vi "Turn Off all Chan.vi"(8 "error in (no error)":errorcluster, 11 "3300 in":refnum<class "3300.lvclass">) -> (0 "error out":errorcluster, 3 "3300 out":refnum<class "3300.lvclass">)   [LabVIEW 2019, in "3300.lvlib" / "3300.lvclass"]
uses:
  Library/3300.lvclass
  C:/Users/Public/Documents/Development/builds/Instruments/Electronic Load.lvlibp/Library/Electronic Load.lvclass
  builds/Instruments/Electronic Load.lvlibp/Custom Controls/E-Load Mode.ctl
  builds/Instruments/Electronic Load.lvlibp/Accessors/Trigger/Read Pulse Enable.vi
  builds/Instruments/Electronic Load.lvlibp/Accessors/Trigger/Read All Pulse.vi
  builds/Instruments/Electronic Load.lvlibp/Library/Electronic Load.lvclass
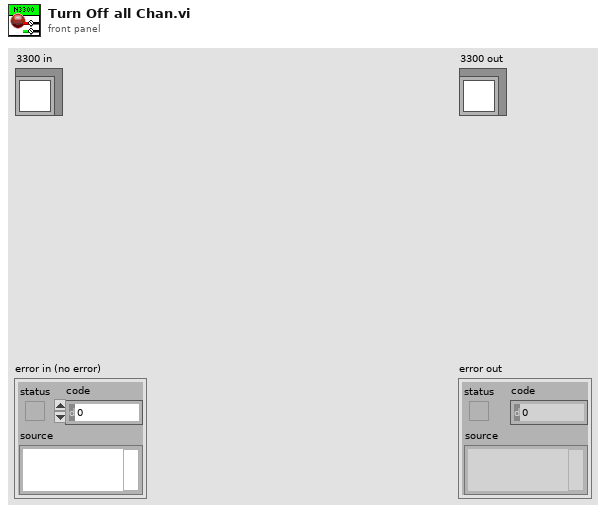
[diagram p1: front panel]
types:
  T1 = typedef "Electronic Load.lvlibp/Electronic Load.lvclass/E-Load Mode.ctl" = enum16{"Current", "Resistance", "Voltage"}
  T2 = typedef "Electronic Load.lvlibp/Electronic Load.lvclass/Trigger Settings.ctl" = cluster{"Mode":T1, "Initial":dbl, "Transient":dbl, "Interval":dbl, "Width":dbl, "Delay":dbl, "Data Pts":i32, "Slew Rate":dbl}
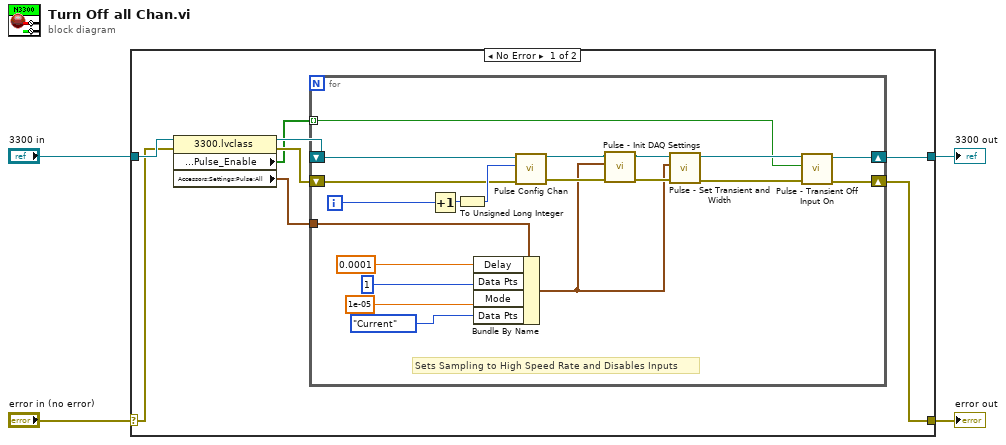
[diagram p0: block diagram]
diagram:
  n1 = case shown="No Error" "error in (no error)" {
    selector: "error in (no error)" -> [w8 w34]
    tunnel: [w7 w34] -> w3
    tunnel: [w9 w33] -> w1
    tunnel: "3300 in" -> [w12 w33]
    frame No Error {
      n2 = property class="3300.lvclass"(reference=w12, error in=w8) -> (reference out=w11:refnum<class "3300.lvclass">, error out=w10:errorcluster, "Accessors:Settings:Pulse:Pulse_Enable"=w5:bool[], "Accessors:Settings:Pulse:All"=w6:T2)
      n3 = for {
        shift-right: [w32] -> w9
        shift-left: w11 -> [w30]
        shift-right: [w31] -> w7
        shift-left: w10 -> [w27]
        tunnel: w6 -> [w20]
        tunnel: w5 -> [w13] mode=indexing
        i -> [w19]
        # "Sets Sampling to High Speed Rate and Disables Inputs"
        n4 = Increment(x=w19) -> (x+1=w29:i32)
        n5 = To Unsigned Long Integer(number=w29) -> (unsigned 32bit integer=w28:u32)
        n6 = Bundle By Name(cluster=w20, "Delay"=0.0001 ("Setting.Trigger Settings.Pulse Width (s)"), "Data Pts"=1 ("Setting.Trigger Settings.Data Points"), "Mode"=1e-05 ("Setting.Trigger Settings.Pulse Width (s)"), "Data Pts"=E-Load_Mode."Current" ("Setting.Trigger Settings.Mode")) -> (w14:T2)
        n7 = call "Pulse Config Chan.vi"("error in (no error)"=w27, "Channel (1)"=w28, "3300 in"=w30) -> ("error out"=w15:errorcluster, "3300 out"=w16:refnum<class "3300.lvclass">)  [unwired: 7 in]
        n8 = call "Pulse - Init DAQ Settings.vi"("error in (no error)"=w15, "Trigger Settings"=w14, "3300 in"=w16) -> ("error out"=w18:errorcluster, "3300 out"=w17:refnum<class "3300.lvclass">)  [unwired: 7 in]
        n9 = call "Pulse - Set Transient and Width.vi"("error in (no error)"=w18, "Trigger Settings"=w14, "3300 in"=w17) -> ("error out"=w25:errorcluster, "3300 out"=w26:refnum<class "3300.lvclass">)  [unwired: 7 in]
        n10 = call "Pulse - Transient Off Input On.vi"("error in (no error)"=w25, "Trig Enable"=w13, "3300 in"=w26) -> ("error out"=w31:errorcluster, "3300 out"=w32:refnum<class "3300.lvclass">)  [unwired: 7 in]
      }
    }
    frame Error {
    }
  }
  "error out" <- w3
  "3300 out" <- w1
